vi "In Range With Tolerance.vi"(0 "Center":dbl, 1 "Tolerance":dbl=0.1, 2 "Value":dbl) -> (5 "In-Range":bool)   [LabVIEW 2010]
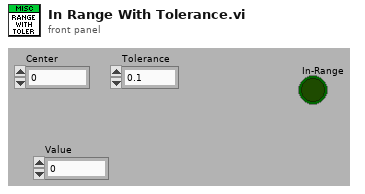
[diagram p1: front panel]
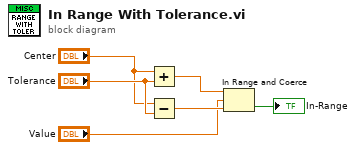
[diagram p0: block diagram]
diagram:
  n1 = Add(x="Center", y="Tolerance") -> (x+y=w2:dbl)
  n2 = Subtract(x="Center", y="Tolerance") -> (x-y=w5:dbl)
  n3 = In Range and Coerce(upper limit=w2, x="Value", lower limit=w5) -> (In Range?=→"In-Range":bool)  [unwired: 1 out]
